vi "dsdll_get_dll_version_string.vi"(8 "error in":errorcluster, 11 "dsdll instance in":T1={"dsdll path"=path "E:/LVprog/DirectSoundDLL/dsdll.dll", "dsdll handle"=[], "output devices"=[], "capture devices"=[]}) -> (0 "error out":errorcluster, 2 "version string":string, 3 "dsdll instance out":T1)   [LabVIEW 2020, in "dsdll.lvlib"]
doc: "Call to get status version string of the 'dsdll.dll' library."
uses:
  dsdll.lvlib
  dsdll_instance.ctl
  dsdll_device_record.ctl
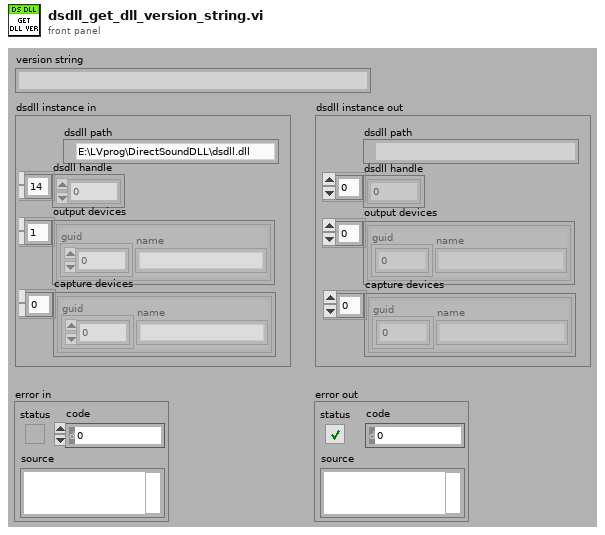
[diagram p1: front panel]
types:
  T1 = typedef "dsdll.lvlib/dsdll_instance.ctl" = cluster{"dsdll path":path, "dsdll handle":u8[], "output devices":T2[], "capture devices":T2[]}
  T2 = typedef "dsdll.lvlib/dsdll_device_record.ctl" = cluster{"guid":u8[], "name":string}
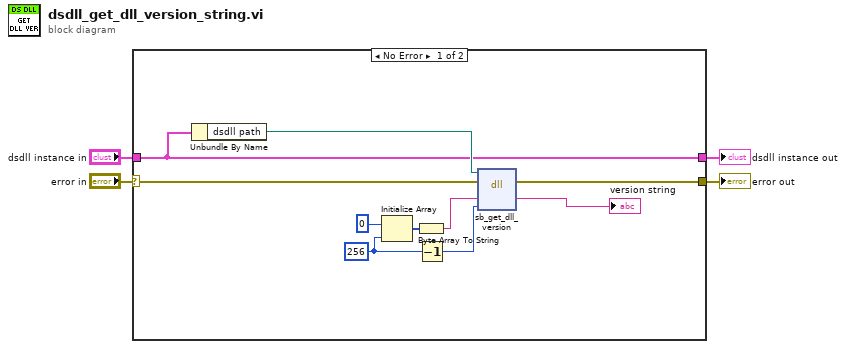
[diagram p0: block diagram]
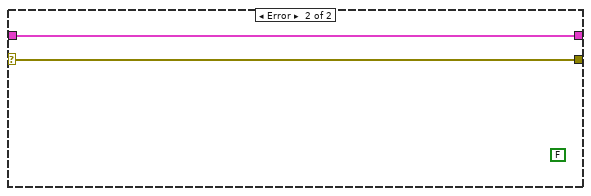
[diagram p2: hidden frame]
diagram:
  n1 = case shown="No Error" "error in" {
    selector: "error in" -> [w12 w15]
    tunnel: "dsdll instance in" -> [w5 w16]
    tunnel: [w13 w15] -> w3
    tunnel: [w5 w16] -> w4
    frame No Error {
      w7 = 256
      n2 = Unbundle By Name(w5) -> ("dsdll path"=w14:path)
      n3 = Initialize Array(u8 0, w7) -> (w9:u8[])
      n4 = Byte Array To String(unsigned byte array=w9) -> (string=w8:string)
      n5 = Decrement(x=w7) -> (x-1=w6:i32)
      n6 = dll-call lib="dsdll.dll" fn="sb_get_dll_version" ("sb_get_handle_size()")(path in=w14, error in=w12, "str"=w8, "maxlen"=w6) -> (error out=w13:errorcluster, "str"=→"version string":string)  [unwired: 3 in, 1 out]
    }
    frame Error {
      (unwired) FALSE
    }
  }
  "error out" <- w3
  "dsdll instance out" <- w4
